vi "Settings - NI 9263.vi"(8 "Error In":errorcluster) -> (0 "Error Out":errorcluster={"status"=TRUE, "code"=-200077, "source"="Property Node DAQmx Channel (arg 2) in DAQmx Create Channel (AI-Temperature-Thermocouple).vi:1->Settings - NI 9211.vi <append>\n<B>Property: </B>AI.Temp.Units\n<B>Requested Value: </B>\n<B>You Can Select: </B>Deg C, Deg F, Kelvins, Deg R, From Custom Scale\n\n<B>Channel Name: </B>Temperature\n\n<B>Task Name: </B>_unnamedTask<E>"}, 3 "Cancelled?":bool)   [LabVIEW 2011]
doc: "This VI will get settings for NI 9211 measurement."
uses:
  SubVIs/Controls/4ch_ao.ctl
  SubVIs/Controls/TransparencyEffectOperations.ctl
  <vilib>/DAQmx/create/channels.llb/DAQmx Create Channel (AO-Voltage-Basic).vi
  <vilib>/DAQmx/configure/timing.llb/DAQmx Timing (Sample Clock).vi
  Program Files/National Instruments/LabVIEW 2011/resource/objmgr/daqmx.rc
panel:
  in  "Channel":T1
  in  "Unit":i32(ring)=10348 items=["Volts"=10348, "From Custom Scale"=10065]
  in  "Terminal Config":i32(ring)=10083 items=["Default"=-1, "RSE"=10083, "Differential"=10106, "Pseudodifferential"=12529]
  in  "Sample Mode":i32(ring)=10123 items=["Finite Samples"=10178, "Continuous Samples"=10123, "Hardware Timed Single Point"=12522]
  in  "Nr of Samples":i32=1000
  in  "Rate":dbl=10000.0
  in  "Min":dbl=-10.0
  in  "Max":dbl=10.0
  in  "Header For Measurement File":string="Voltage"
  in  "Cancel Button":bool
  in  "OK Button":bool
  # "NI 9263"
  # "Meas File Settings"
  # "Hardware Settings"
  # "Signal Output Range"
  # "Scaled Units"
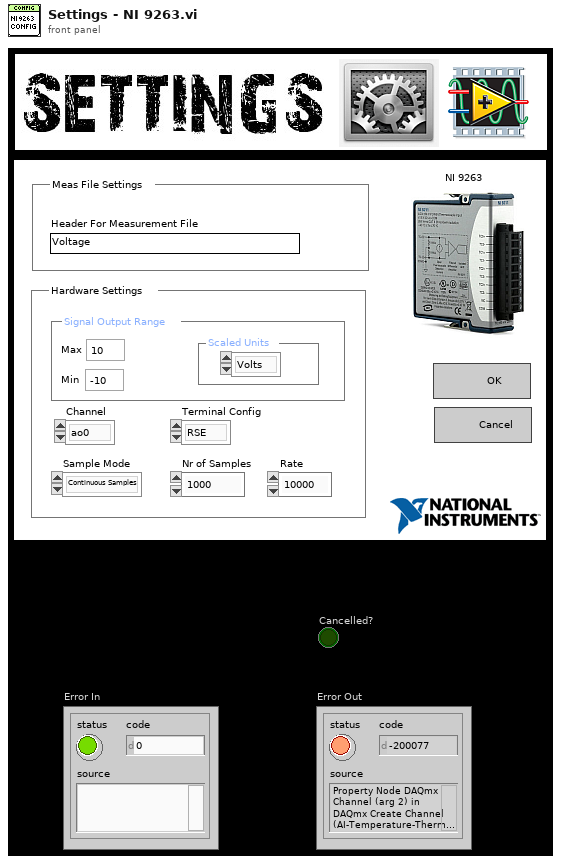
[diagram p1: front panel]
types:
  T1 = typedef "4ch_ao.ctl" = enum16{"ao0", "ao1", "ao2", "ao3"}
  T2 = typedef "TransparencyEffectOperations.ctl" = enum16{"Show", "Hide 80%", "Hide All"}
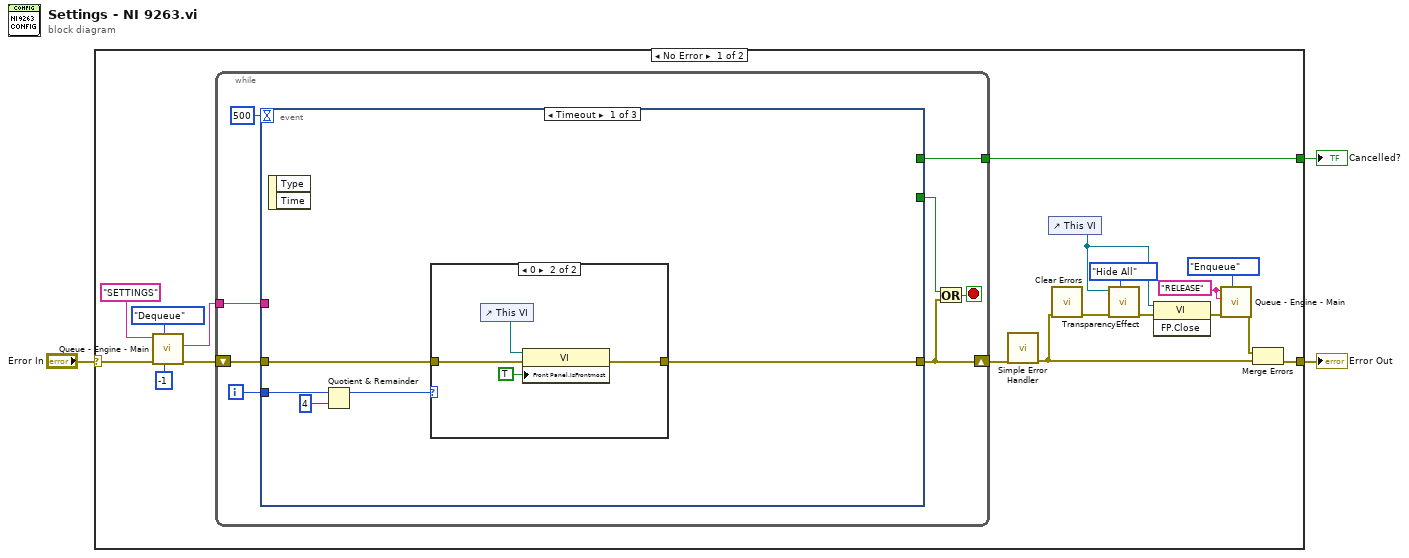
[diagram p0: block diagram]
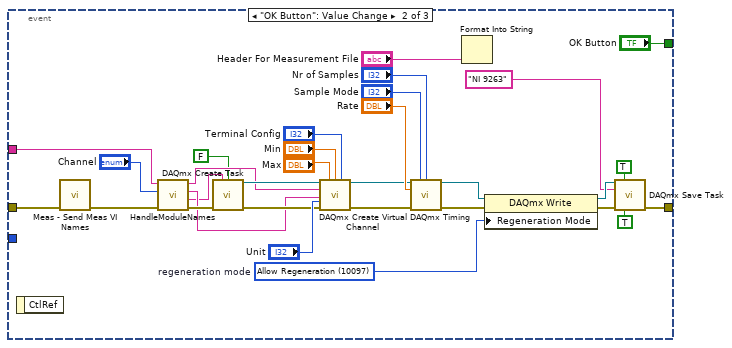
[diagram p3: hidden frame]
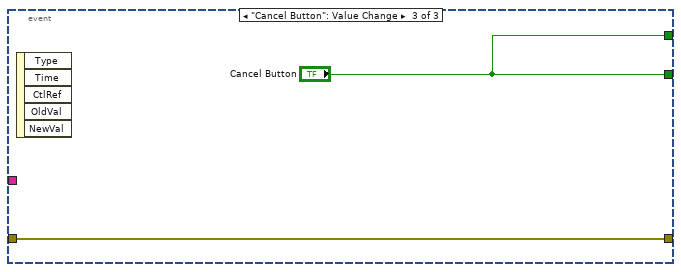
[diagram p4: hidden frame]
diagram:
  n1 = case shown="No Error" "Error In" {
    selector: "Error In" -> [w18 w73]
    tunnel: [w21 _] -> w3
    tunnel: [w4 w73] -> w2
    frame No Error {
      w10 = "RELEASE" ("Queue Data In")
      n2 = call "Queue - Engine - Main.vi"("timeout in ms (-1)"=-1, "Operation"=enum16{"Enqueue", "Dequeue", "Flush", "Release"}."Dequeue", "error in"=w18, "Queue Name In"="SETTINGS") -> ("error out"=w17:errorcluster, "Data Out"=w16:string)  [unwired: 5 in, 1 out]
      n3 = while {
        tunnel: [w29] -> w21
        shift-right: [w24] -> w5
        shift-left: w17 -> [w28]
        tunnel: w16 -> [w27]
        i -> [w25]
        stop <- w22 stop-if-true
        n4 = event shown="[0] Timeout" {
          selector: _ -> [_ _ _]
          dyn-events: _ -> [_ _ _]
          timeout: 500 -> [_ _ _]
          tunnel: [_ "OK Button" "Cancel Button"] -> w23
          tunnel: [_ _ "Cancel Button"] -> w29
          tunnel: [w33 w43 w71] -> w24
          tunnel: w28 -> [w34 w47 w71]
          tunnel: w27 -> [_ w48 _]
          tunnel: w25 -> [w32 _ _]
          event Timeout {
            n5 = event-data() -> ()  [unwired: 1 in, 2 out]
            n6 = Quotient & Remainder(x=w32, y=4) -> (x-y*floor(x/y)=w30:i32)  [unwired: 1 out]
            n7 = case shown="0" w30 {
              tunnel: w34 -> [w35 w38]
              tunnel: [w35 w37] -> w33
              frame Default {
              }
              frame 0 {
                n8 = control-ref of="This VI"() -> (w39:refnum<vi>)
                n9 = property class="VI"(reference=w39, error in=w38, "Front Panel.IsFrontmost"=TRUE ("Front Panel Window:Is Frontmost")) -> (error out=w37:errorcluster)  [unwired: 1 out]
              }
            }
          }
          event "OK Button": Value Change {
            w66 = 10097 items=["Allow Regeneration"=10097, "Do Not Allow Regeneration"=10158]  # regeneration mode
            n10 = event-data() -> ()  [unwired: 1 in, 1 out]
            n11 = call "Meas - Send Meas VI Names.vi"("Error In"=w47) -> ("Error Out"=w46:errorcluster)  [unwired: 10 in]
            n12 = call "HandleModuleNames.vi"("Error In"=w46, "Channel"="Channel", "Data In"=w48) -> ("Error Out"=w53:errorcluster, "Module and CH 2"=w49:string, "Module and CH"=w51:string, "Channel"=w54:string)  [unwired: 5 in]
            n13 = call <vilib>:"DAQmx Create Task.vi"("new task name"=w49, "auto cleanup"=FALSE, "error in"=w53) -> ("task out"=w56:refnum<k21>, "error out"=w55:errorcluster)  [unwired: 11 in]
            n14 = call-poly <vilib>:"DAQmx Create Virtual Channel.vi"("task in"=w56, "maximum value"="Max", "minimum value"="Min", "output terminal configuration"="Terminal Config", "physical channels"=w54, "name to assign"=w51, "units"="Unit", "error in"=w55) -> ("task out"=w58:refnum<k21>, "error out"=w59:errorcluster)  [unwired: 2 in, 4 out]
            n15 = call-poly <vilib>:"DAQmx Timing.vi"("task/channels in"=w58, "sample mode"="Sample Mode", "samples per channel"="Nr of Samples", "rate"="Rate", "error in"=w59) -> ("task out"=w65:refnum<k21>, "error out"=w64:errorcluster)  [unwired: 2 in, 7 out]
            n16 = Format Into String("Header For Measurement File") -> ()  [unwired: 3 in, 2 out]
            n17 = property class="DAQmx Write"(reference=w65, error in=w64, "Regeneration Mode"=w66) -> (reference out=w41:refnum<k21>, error out=w42:errorcluster)
            n18 = call <vilib>:"DAQmx Save Task.vi"("task/channels in"=w41, "allow interactive editing?"=TRUE, "save as"="NI 9263" ("format string"), "error in"=w42, "overwrite existing task?"=TRUE) -> ("error out"=w43:errorcluster)  [unwired: 9 in, 1 out]
          }
          event "Cancel Button": Value Change {
            n19 = event-data() -> ()  [unwired: 1 in, 5 out]
          }
        }
        n20 = Or(x=w23, y=w24) -> (x .or. y?=w22:bool)
      }
      n21 = call <vilib>:"Simple Error Handler.vi"("error in (no error)"=w5) -> ("error out"=w7:errorcluster)  [unwired: 4 in, 4 out]
      n22 = control-ref of="This VI"() -> (w14:refnum<vi>)
      n23 = call <vilib>:"Clear Errors.vi"("error in (no error)"=w7) -> ("error out"=w6:errorcluster)  [unwired: 6 in]
      n24 = call "TransparencyEffect.vi"("Operation"=TransparencyEffectOperations."Hide All", "error in"=w6, "VI Ref in"=w14) -> ("error out"=w11:errorcluster)  [unwired: 8 in]
      n25 = invoke class="VI" method="FP.Close"(reference=w14, error in=w11) -> (error out=w8:errorcluster)  [unwired: 1 in, 2 out]
      n26 = call "Queue - Engine - Main.vi"("Operation"=enum16{"Enqueue", "Dequeue", "Flush", "Release"}."Enqueue", "error in"=w8, "Queue Data In"=w10, "Queue Name In"=w10) -> ("error out"=w9:errorcluster)  [unwired: 5 in, 2 out]
      n27 = Merge Errors(w9, w7) -> (w4:errorcluster)
    }
    frame Error {
    }
  }
  "Cancelled?" <- w3
  "Error Out" <- w2
